vi "Dual_DM_Control_Main_V2.vi"() -> ()   [LabVIEW 2014]
uses:
  Controls/MirrorModes.ctl
  Controls/Standard Action.ctl
  <vilib>/Analysis/baseanly.llb/Mean (DBL).vi
  <vilib>/Utility/file.llb/Read From Spreadsheet File (DBL).vi
  <vilib>/Analysis/NI_AALBase.lvlib
  <vilib>/Utility/file.llb/Write To Spreadsheet File (DBL).vi
panel:
  in  "Active Mirror":enum32{"Mirror 1", "Mirror 2"}(radio)
  in  "Clear Modes":bool
  in  "Mirror Modes":T1
  in  "Load Modes":bool
  in  "Save Modes":bool
  in  "Scan Modes":bool
  in  "Load Flat":bool
  in  "Apply Zero":bool
  in  "Load V Map":bool
  in  "Save V Map":bool
  in  "Apply Flat":bool
  in  "Center Bias":bool
  in  "Exit":bool
  out "Pixel Map (-1 to 1)":dbl[][](graph)
  # "Mode"
  # "Amount (nm)"
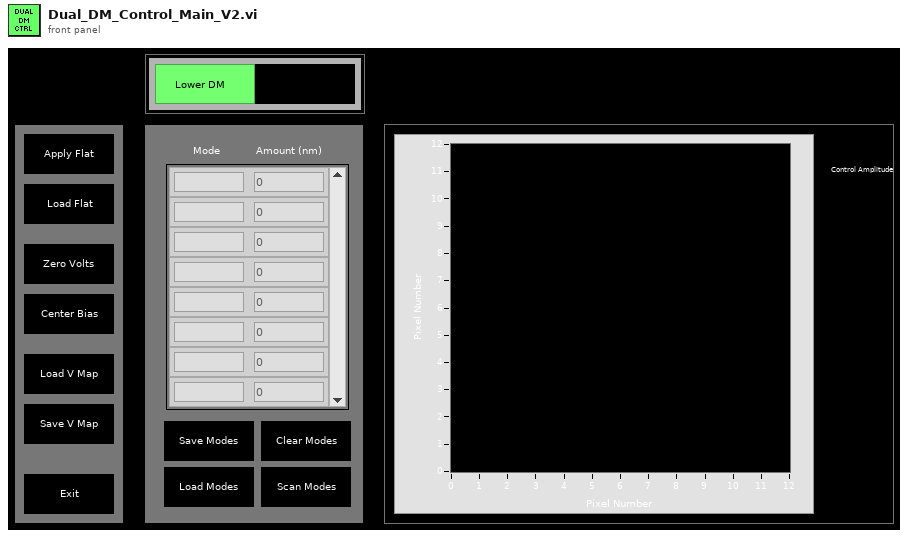
[diagram p1: front panel]
types:
  T1 = typedef "MirrorModes.ctl" = cluster{"Mode":string, "Amplitude":dbl}[]
  T2 = typedef "Standard Action.ctl" = enum16{"Read", "Write"}
  T3 = typedef "MirrorModes_DUAL.ctl" = cluster{"Mode":string, "Amplitude":dbl}[][]
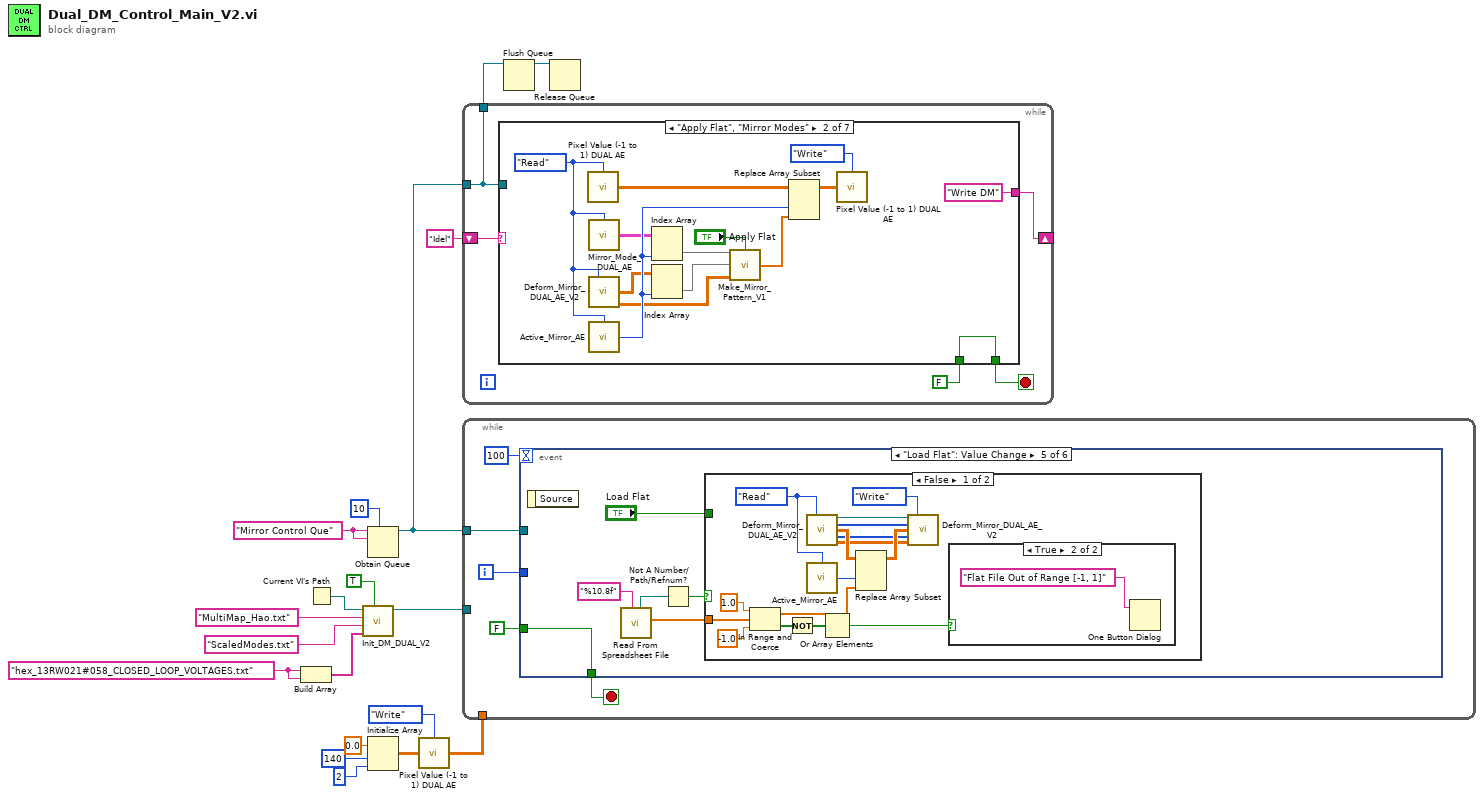
[diagram p0: block diagram]
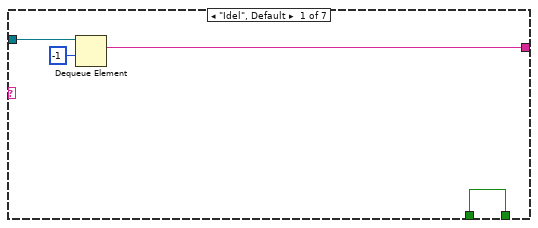
[diagram p2: hidden frame]
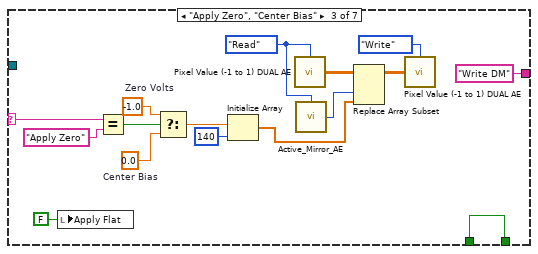
[diagram p3: hidden frame]
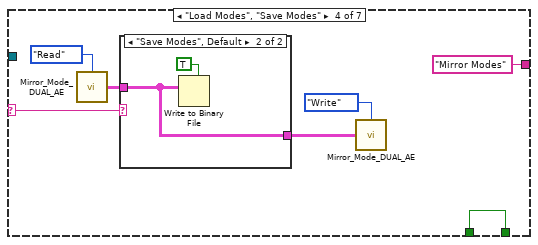
[diagram p4: hidden frame]
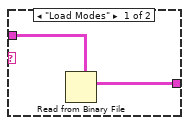
[diagram p5: hidden frame]
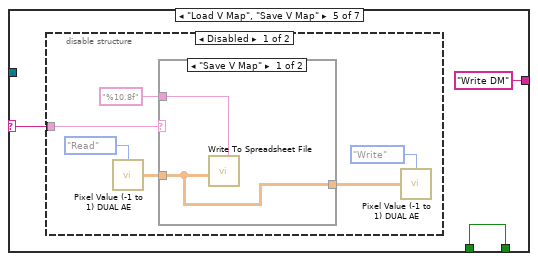
[diagram p6: hidden frame]
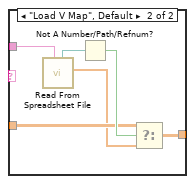
[diagram p7: hidden frame]
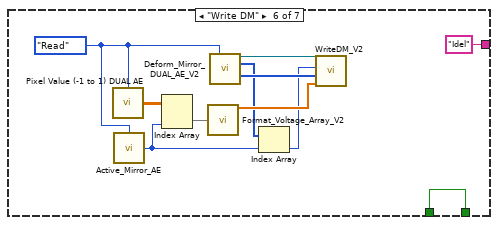
[diagram p9: hidden frame]
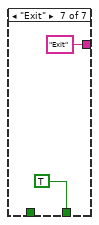
[diagram p10: hidden frame]
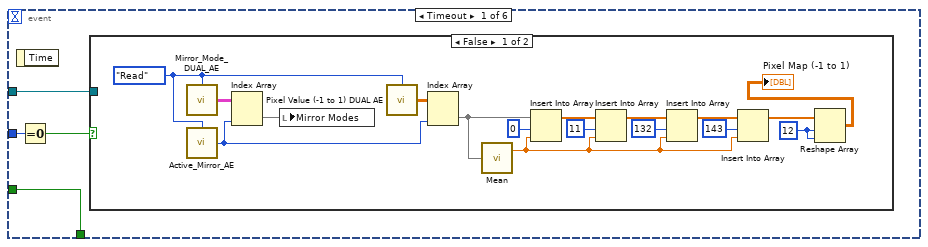
[diagram p11: hidden frame]
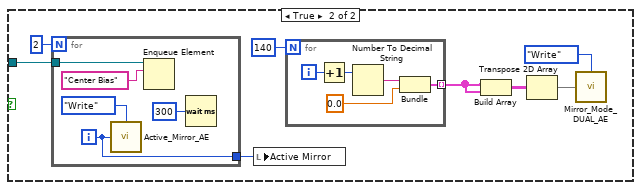
[diagram p12: hidden frame]
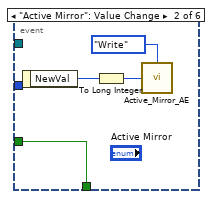
[diagram p13: hidden frame]
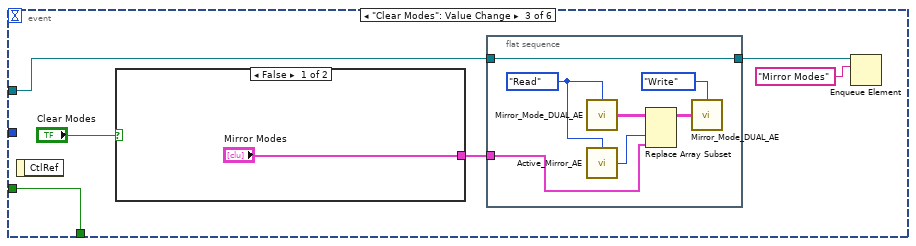
[diagram p14: hidden frame]
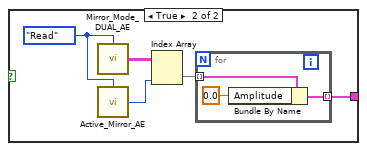
[diagram p15: hidden frame]
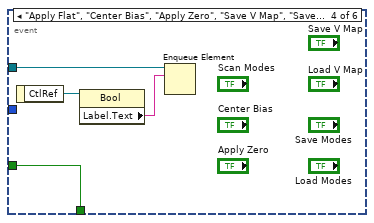
[diagram p16: hidden frame]
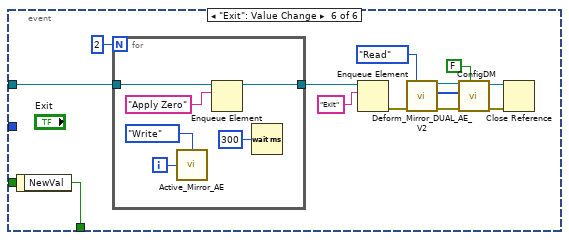
[diagram p19: hidden frame]
diagram:
  w8 = "hex_13RW021#058_CLOSED_LOOP_VOLTAGES.txt" ("name or relative path")
  w19 = "Mirror Control Que" ("name (unnamed)")
  n1 = Build Array(w8, w8) -> (w7:string[])
  n2 = Current VI's Path() -> (path=w11:path)
  n3 = call "Init_DM_DUAL_V2.vi"("BM Flat"=TRUE, "BM Flat File"=w7, "Mirror Modes File"="ScaledModes.txt" ("name or relative path"), "DM Mapping File"="MultiMap_Hao.txt" ("name or relative path"), "Base File Path"=w11) -> ("reference out"=w17:refnum<k7>)  [unwired: 6 in]
  n4 = Obtain Queue(max queue size (-1, unlimited)=10, name (unnamed)=w19, element data type=w19) -> (queue out=w13:refnum<queue>)  [unwired: 2 in, 2 out]
  n5 = Initialize Array(0.0 ("element"), 140 ("dimension size"), 2 ("dimension size")) -> (w3:dbl[][])
  n6 = call "Pixel Value (-1 to 1) DUAL AE.vi"("Action"=Standard_Action."Write", "Pixel Value (-1 to 1)"=w3) -> ("Pixel Value (-1 to 1) Out"=w1:dbl[][])  [unwired: 13 in]
  n7 = while {
    tunnel: w13 -> [w20]
    shift-right: [w24] -> _
    shift-left: "Idel" ("name (unnamed)") -> [w23]
    tunnel: [w20] -> w16
    stop <- w22 stop-if-true
    n8 = case shown="\"Apply Flat\", \"Mirror Modes\"" w23 {
      selector: w23 -> [_ _ w54 w61 w71 _ _]
      tunnel: w20 -> [w28 _ _ _ _ _ _]
      tunnel: [w26 "Write DM" ("name (unnamed)") "Write DM" ("name (unnamed)") "Mirror Modes" ("name (unnamed)") "Write DM" ("name (unnamed)") "Idel" ("name (unnamed)") "Exit" ("name (unnamed)")] -> w24
      tunnel: [w25 w41 w58 w65 w72 w97 TRUE] -> w22
      tunnel: FALSE -> [w25 w41 w58 w65 w72 w97 _]
      frame "Idel", Default {
        n9 = Dequeue Element(queue=w28, timeout in ms (-1)=-1) -> (element=w26:string)  [unwired: 1 in, 3 out]
      }
      frame "Apply Flat", "Mirror Modes" {
        w36 = Standard_Action."Read" ("Action")
        n10 = call "Pixel Value (-1 to 1) DUAL AE.vi"("Action"=w36) -> ("Pixel Value (-1 to 1) Out"=w37:dbl[][])  [unwired: 14 in]
        n11 = call "Mirror_Mode_DUAL_AE.vi"("Action"=w36) -> ("Mirror Modes Out"=w33:T3)  [unwired: 14 in]
        n12 = call "Deform_Mirror_DUAL_AE_V2.vi"("Action"=w36) -> ("Flat Files Out"=w31:dbl[][], "Mode Matrix Out"=w30:dbl[][])  [unwired: 10 in, 3 out]
        n13 = call "Active_Mirror_AE.vi"("Action"=w36) -> ("Active Mirror"=w39:i32)  [unwired: 14 in]
        n14 = Index Array(array=w33, index (col)=w39) -> (element=w34:cluster{"Mode":string, "Amplitude":dbl}[])  [unwired: 1 in]
        n15 = Index Array(array=w31, index (col)=w39) -> (element=w32:dbl[])  [unwired: 1 in]
        n16 = call "Make_Mirror_Pattern_V1.vi"("Mirror Modes In"=w34, "Flat On?"="Apply Flat", "Flat File In"=w32, "Mirror Modes Array"=w30) -> ("Pixel Value U (-1 to 1)"=w38:dbl[])  [unwired: 11 in]
        n17 = Replace Array Subset(array=w37, new element=w38, index (col)=w39) -> (w40:dbl[][])  [unwired: 1 in]
        n18 = call "Pixel Value (-1 to 1) DUAL AE.vi"("Action"=Standard_Action."Write", "Pixel Value (-1 to 1)"=w40) -> ()  [unwired: 13 in, 1 out]
      }
      frame "Apply Zero", "Center Bias" {
        w46 = Standard_Action."Read" ("Action")
        w50 = -1.0  # Zero Volts
        w52 = 0.0  # Center Bias
        n19 = local write "Apply Flat"(FALSE ("Apply Flat")) -> ()
        n20 = Equal?(x=w54, y="Apply Zero") -> (x = y?=w53:bool)
        n21 = Select(t=w50, s=w53, f=w52) -> (s? t:f=w51:dbl)
        n22 = Initialize Array(w51, 140 ("dimension size")) -> (w43:dbl[])
        n23 = call "Pixel Value (-1 to 1) DUAL AE.vi"("Action"=w46) -> ("Pixel Value (-1 to 1) Out"=w44:dbl[][])  [unwired: 14 in]
        n24 = call "Active_Mirror_AE.vi"("Action"=w46) -> ("Active Mirror"=w45:i32)  [unwired: 14 in]
        n25 = Replace Array Subset(array=w44, new element=w43, index (col)=w45) -> (w48:dbl[][])  [unwired: 1 in]
        n26 = call "Pixel Value (-1 to 1) DUAL AE.vi"("Action"=Standard_Action."Write", "Pixel Value (-1 to 1)"=w48) -> ()  [unwired: 13 in, 1 out]
      }
      frame "Load Modes", "Save Modes" {
        n27 = call "Mirror_Mode_DUAL_AE.vi"("Action"=Standard_Action."Read") -> ("Mirror Modes Out"=w60:T3)  [unwired: 14 in]
        n28 = case shown="\"Save Modes\", Default" w61 {
          tunnel: w60 -> [w67 w68]
          tunnel: [w66 w68] -> w59
          frame "Load Modes" {
            n29 = Read from Binary File(5:w67) -> (2:w66:T3)  [unwired: 5 in, 3 out]
          }
          frame "Save Modes", Default {
            n30 = Write to Binary File(data=w68, 5:TRUE ("prepend array or string size? (T)")) -> ()  [unwired: 4 in, 3 out]
          }
        }
        n31 = call "Mirror_Mode_DUAL_AE.vi"("Action"=Standard_Action."Write", "Mirror Modes In"=w59) -> ()  [unwired: 13 in, 1 out]
      }
      frame "Load V Map", "Save V Map" {
        n32 = disable-structure shown="Disabled" {
          disable-tunnel: w71 -> [w78 _]
          frame Disabled {
            n33 = call "Pixel Value (-1 to 1) DUAL AE.vi"("Action"=Standard_Action."Read") -> ("Pixel Value (-1 to 1) Out"=w76:dbl[][])  [unwired: 14 in]
            n34 = case shown="\"Save V Map\"" w78 {
              tunnel: w76 -> [w79 w83]
              tunnel: "%10.8f" -> [w80 w86]
              tunnel: [w79 w81] -> w73
              frame "Save V Map" {
                n35 = call-poly <vilib>:"Write To Spreadsheet File.vi"("format (%.3f)"=w80, "1D data"=w79) -> ()  [unwired: 6 in, 1 out]
              }
              frame "Load V Map", Default {
                n36 = call-poly <vilib>:"Read From Spreadsheet File.vi"("format (%.3f)"=w86) -> ("first row"=w82:dbl[], "new file path (Not A Path if cancelled)"=w85:path)  [unwired: 6 in, 3 out]
                n37 = Not A Number/Path/Refnum?(number/path/refnum=w85) -> (NaN/Path/Refnum?=w84:bool)
                n38 = Select(t=w83, s=w84, f=w82) -> (s? t:f=w81:dbl[][])
              }
            }
            n39 = call "Pixel Value (-1 to 1) DUAL AE.vi"("Action"=Standard_Action."Write", "Pixel Value (-1 to 1)"=w73) -> ()  [unwired: 13 in, 1 out]
          }
          frame Enabled {
          }
        }
      }
      frame "Write DM" {
        w90 = Standard_Action."Read" ("Action")
        n40 = call "Pixel Value (-1 to 1) DUAL AE.vi"("Action"=w90) -> ("Pixel Value (-1 to 1) Out"=w92:dbl[][])  [unwired: 14 in]
        n41 = call "Active_Mirror_AE.vi"("Action"=w90) -> ("Active Mirror"=w88:i32)  [unwired: 14 in]
        n42 = Index Array(array=w92, index (col)=w88) -> (element=w91:dbl[])  [unwired: 1 in]
        n43 = call "Format_Voltage_Array_V2.vi"("Pixel Level (-1 to 1)"=w91) -> ("Voltage Array (Volts)"=w93:dbl[])  [unwired: 13 in, 1 out]
        n44 = call "Deform_Mirror_DUAL_AE_V2.vi"("Action"=w90) -> ("Refnum Out"=w95:refnum<k7>, "IDs Out"=w89:i32[], "Multi Map Data Out"=w94:i32[])  [unwired: 10 in, 2 out]
        n45 = Index Array(array=w89, index=w88) -> (element=w87:i32)
        n46 = call "WriteDM_V2.vi"("reference in"=w95, "nDevId"=w87, "MultiDM  Mapping"=w94, "Voltage Array in"=w93) -> ()  [unwired: 2 in, 2 out]
      }
      frame "Exit" {
      }
    }
  }
  n47 = while {
    tunnel: w13 -> [w100]
    tunnel: w17 -> [_]
    tunnel: w1 -> [_]
    i -> [w101]
    stop <- w104 stop-if-true
    n48 = event shown="[4] \"Load Flat\": Value Change" {
      selector: _ -> [_ _ _ _ _ _]
      dyn-events: _ -> [_ _ _ _ _ _]
      timeout: 100 -> [_ _ _ _ _ _]
      tunnel: [w108 w147 w153 w173 w179 w208] -> w104
      tunnel: FALSE -> [w108 w147 w153 w173 w179 _]
      tunnel: w101 -> [w107 _ _ _ _ _]
      tunnel: w100 -> [w105 _ w152 w172 _ w206]
      event Timeout {
        n49 = event-data() -> ()  [unwired: 1 in, 1 out]
        n50 = Equal To 0?(x=w107) -> (x = 0?=w106:bool)
        n51 = case shown="False" w106 {
          tunnel: w105 -> [_ w133]
          frame False {
            w121 = 12 ("dimension size")
            w122 = Standard_Action."Read" ("Action")
            n52 = call "Mirror_Mode_DUAL_AE.vi"("Action"=w122) -> ("Mirror Modes Out"=w109:T3)  [unwired: 14 in]
            n53 = call "Active_Mirror_AE.vi"("Action"=w122) -> ("Active Mirror"=w124:i32)  [unwired: 14 in]
            n54 = Index Array(array=w109, index (col)=w124) -> (element=w110:cluster{"Mode":string, "Amplitude":dbl}[])  [unwired: 1 in]
            n55 = local write "Mirror Modes"(w110) -> ()
            n56 = call "Pixel Value (-1 to 1) DUAL AE.vi"("Action"=w122) -> ("Pixel Value (-1 to 1) Out"=w123:dbl[][])  [unwired: 14 in]
            n57 = Index Array(array=w123, index (col)=w124) -> (element=w125:dbl[])  [unwired: 1 in]
            n58 = call-poly <vilib>:"Mean.vi"("X"=w125) -> ("mean"=w119:dbl)  [unwired: 1 out]
            n59 = Insert Into Array(array=w125, index=0, new element=w119) -> (w114:dbl[])
            n60 = Insert Into Array(array=w114, index=11, new element=w119) -> (w116:dbl[])
            n61 = Insert Into Array(array=w116, index=132, new element=w119) -> (w118:dbl[])
            n62 = Insert Into Array(array=w118, index=143, new element=w119) -> (w111:dbl[])
            n63 = Reshape Array(w111, w121, w121) -> (→"Pixel Map (-1 to 1)":dbl[][])
          }
          frame True {
            n64 = for {
              N: 2 -> [_]
              tunnel: w133 -> [w138]
              tunnel: [w134] -> w126
              i -> [w134]
              n65 = call "Active_Mirror_AE.vi"("Action"=Standard_Action."Write", "Active Mirror In"=w134) -> ()  [unwired: 13 in, 1 out]
              n66 = Enqueue Element(queue=w138, element="Center Bias") -> ()  [unwired: 2 in, 3 out]
              n67 = Wait (ms)(milliseconds to wait=u32 300) -> ()  [unwired: 1 out]
            }
            n68 = local write "Active Mirror"(w126) -> ()
            n69 = for {
              N: 140 -> [_]
              tunnel: [w139] -> w130 mode=indexing
              i -> [w143]
              n70 = Increment(x=w143) -> (x+1=w142:i32)
              n71 = Number To Decimal String(number=w142) -> (decimal integer string=w141:string)  [unwired: 1 in]
              n72 = Bundle(w141, 0.0) -> (w139:cluster{string, dbl})  [unwired: 1 in]
            }
            n73 = Build Array(w130, w130) -> (w128:cluster{string, dbl}[][])
            n74 = Transpose 2D Array(2D array=w128) -> (transposed array=w127:cluster{string, dbl}[][])
            n75 = call "Mirror_Mode_DUAL_AE.vi"("Action"=Standard_Action."Write", "Mirror Modes In"=w127) -> ()  [unwired: 13 in, 1 out]
          }
        }
      }
      event "Active Mirror": Value Change {
        n76 = event-data() -> ("NewVal"=w146:enum32{"Mirror 1", "Mirror 2"})  [unwired: 1 in]
        n77 = To Long Integer(number=w146) -> (32bit integer=w145:i32)
        n78 = call "Active_Mirror_AE.vi"("Action"=Standard_Action."Write", "Active Mirror In"=w145) -> ()  [unwired: 13 in, 1 out]
      }
      event "Clear Modes": Value Change {
        n79 = event-data() -> ()  [unwired: 1 in, 1 out]
        n80 = case shown="False" "Clear Modes" {
          tunnel: ["Mirror Modes" w155] -> w148
          frame False {
          }
          frame True {
            w158 = Standard_Action."Read" ("Action")
            n81 = call "Mirror_Mode_DUAL_AE.vi"("Action"=w158) -> ("Mirror Modes Out"=w157:T3)  [unwired: 14 in]
            n82 = call "Active_Mirror_AE.vi"("Action"=w158) -> ("Active Mirror"=w159:i32)  [unwired: 14 in]
            n83 = Index Array(array=w157, index (col)=w159) -> (element=w156:cluster{"Mode":string, "Amplitude":dbl}[])  [unwired: 1 in]
            n84 = for {
              tunnel: w156 -> [w162] mode=indexing
              tunnel: [w160] -> w155 mode=indexing
              n85 = Bundle By Name(cluster=w162, "Amplitude"=0.0) -> (w160:cluster{"Mode":string, "Amplitude":dbl})
            }
          }
        }
        n86 = flat-sequence {
          tunnel: w148 -> [w163]
          tunnel: w152 -> [w169]
          tunnel: [w169] -> w150
          frame #0 {
            w166 = Standard_Action."Read" ("Action")
            n87 = call "Mirror_Mode_DUAL_AE.vi"("Action"=w166) -> ("Mirror Modes Out"=w165:T3)  [unwired: 14 in]
            n88 = call "Active_Mirror_AE.vi"("Action"=w166) -> ("Active Mirror"=w167:i32)  [unwired: 14 in]
            n89 = Replace Array Subset(array=w165, new element=w163, index (col)=w167) -> (w168:T3)  [unwired: 1 in]
            n90 = call "Mirror_Mode_DUAL_AE.vi"("Action"=Standard_Action."Write", "Mirror Modes In"=w168) -> ()  [unwired: 13 in, 1 out]
          }
        }
        n91 = Enqueue Element(queue=w150, element="Mirror Modes") -> ()  [unwired: 2 in, 3 out]
      }
      event "Apply Flat", "Center Bias", "Apply Zero", "Save V Map", "Save Modes", "Load Modes", "Load V Map", "Scan Modes": Value Change {
        n92 = event-data() -> ("CtlRef"=w171:refnum<vi>)  [unwired: 1 in]
        n93 = property class="Bool"(reference=w171) -> ("Label.Text"=w170:string)  [unwired: 1 in, 2 out]
        n94 = Enqueue Element(queue=w172, element=w170) -> ()  [unwired: 2 in, 3 out]
      }
      event "Load Flat": Value Change {
        n95 = event-data() -> ()  [unwired: 1 in, 1 out]
        n96 = call-poly <vilib>:"Read From Spreadsheet File.vi"("format (%.3f)"="%10.8f") -> ("first row"=w175:dbl[], "new file path (Not A Path if cancelled)"=w177:path)  [unwired: 6 in, 3 out]
        n97 = Not A Number/Path/Refnum?(number/path/refnum=w177) -> (NaN/Path/Refnum?=w176:bool)
        n98 = case shown="False" w176 {
          tunnel: w175 -> [w195 _]
          tunnel: "Load Flat" -> [_ _]
          frame False {
            w186 = Standard_Action."Read" ("Action")
            n99 = In Range and Coerce(upper limit=1.0, x=w195, lower limit=-1.0) -> (coerced(x)=w180:dbl[], In Range?=w192:bool[])
            n100 = Not(x=w192) -> (.not. x?=w191:bool[])
            n101 = call "Deform_Mirror_DUAL_AE_V2.vi"("Action"=w186) -> ("Refnum Out"=w181:refnum<k7>, "IDs Out"=w182:i32[], "Flat Files Out"=w187:dbl[][], "Multi Map Data Out"=w183:i32[], "Mode Matrix Out"=w184:dbl[][])  [unwired: 10 in]
            n102 = call "Active_Mirror_AE.vi"("Action"=w186) -> ("Active Mirror"=w189:i32)  [unwired: 14 in]
            n103 = Or Array Elements(Boolean array=w191) -> (logical OR=w190:bool)
            n104 = Replace Array Subset(array=w187, new element=w180, index (col)=w189) -> (w188:dbl[][])  [unwired: 1 in]
            n105 = call "Deform_Mirror_DUAL_AE_V2.vi"("Refnum In"=w181, "Action"=Standard_Action."Write", "IDs In"=w182, "Flat Files In"=w188, "Multi Map Data In"=w183, "Mode Matrix"=w184) -> ()  [unwired: 5 in, 5 out]
            n106 = case shown="True" w190 {
              frame False {
              }
              frame True {
                n107 = One Button Dialog(message="Flat File Out of Range [-1, 1]") -> ()  [unwired: 1 in, 1 out]
              }
            }
          }
          frame True {
          }
        }
      }
      event "Exit": Value Change {
        n108 = event-data() -> ("NewVal"=w208:bool)  [unwired: 1 in]
        n109 = for {
          N: 2 -> [_]
          tunnel: w206 -> [w214]
          tunnel: [w209] -> w197
          i -> [w210]
          n110 = call "Active_Mirror_AE.vi"("Action"=Standard_Action."Write", "Active Mirror In"=w210) -> ()  [unwired: 13 in, 1 out]
          n111 = Enqueue Element(queue=w214, element="Apply Zero") -> (queue out=w209:refnum<queue>)  [unwired: 2 in, 2 out]
          n112 = Wait (ms)(milliseconds to wait=u32 300) -> ()  [unwired: 1 out]
        }
        n113 = Enqueue Element(queue=w197, element="Exit") -> (error out=w201:errorcluster)  [unwired: 2 in, 2 out]
        n114 = call "Deform_Mirror_DUAL_AE_V2.vi"("Action"=Standard_Action."Read") -> ("Refnum Out"=w204:refnum<k7>, "IDs Out"=w199:i32[])  [unwired: 10 in, 3 out]
        n115 = call "ConfigDM.vi"("High Voltage"=FALSE, "error in (no error)"=w201, "Dev IDs"=w199, "Automation Refnum in"=w204) -> ("error out"=w200:errorcluster, "Automation Refnum out"=w203:refnum<k7>)  [unwired: 6 in]
        n116 = Close Reference(reference=w203, error in (no error)=w200) -> ()  [unwired: 1 out]
      }
    }
  }
  n117 = Flush Queue(queue=w16) -> (queue out=w15:refnum<queue>)  [unwired: 1 in, 2 out]
  n118 = Release Queue(queue=w15) -> ()  [unwired: 2 in, 3 out]
